vi "Util_Convert Boolean to String.vi"(4 "Boolean":bool) -> (1 "String":string)   [LabVIEW 2016]
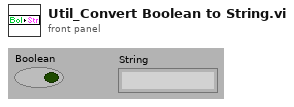
[diagram p1: front panel]
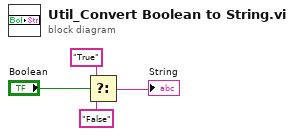
[diagram p0: block diagram]
diagram:
  n1 = Select(t="True", s="Boolean", f="False") -> (s? t:f=→"String":string)
